vi "Sensor List DAO.vi"(7 "refnum":T1, 8 "error in (no error)":errorcluster, 10 "Sensor List In":refnum<class "Sensor List Class.lvclass">, 11 "Actions":T2) -> (0 "error out":errorcluster, 2 "Sensor List Out":refnum<class "Sensor List Class.lvclass">, 4 "refnum out":T1)   [LabVIEW 2013]
uses:
  Metadata/Persistant DAO Actions.ctl
  Sensor List Class.lvclass
  <vilib>/Utility/config.llb/Config Data RefNum.ctl
  <vilib>/Utility/config.llb/NI_LVConfig.lvlib
panel:
  out "Names":string[](array[string])
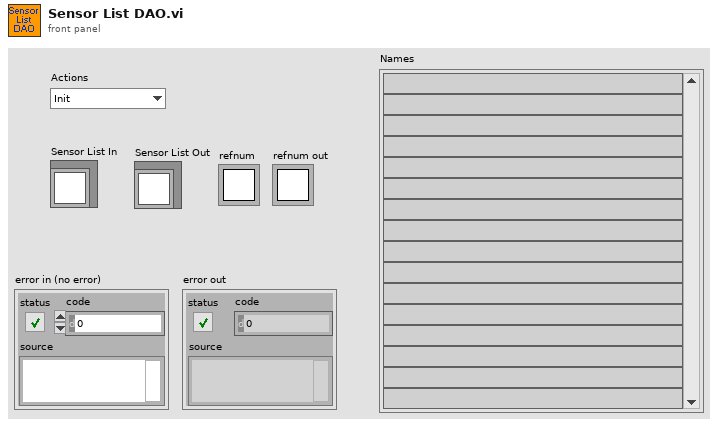
[diagram p1: front panel]
types:
  T1 = typedef "NI_LVConfig.lvlib/Config Data RefNum.ctl" = refnum<k1>
  T2 = typedef "Persistant DAO Actions.ctl" = enum16{"Init", "Get", "Set", "Load", "Save"}
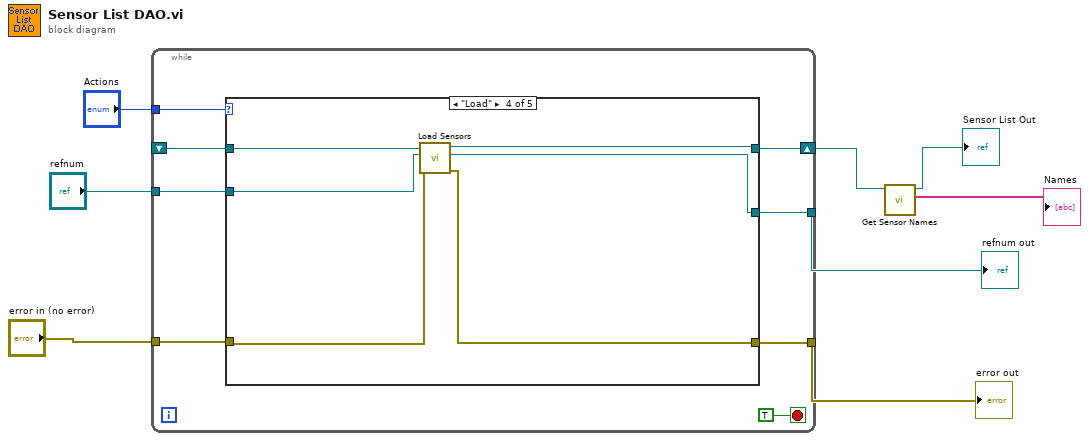
[diagram p0: block diagram]
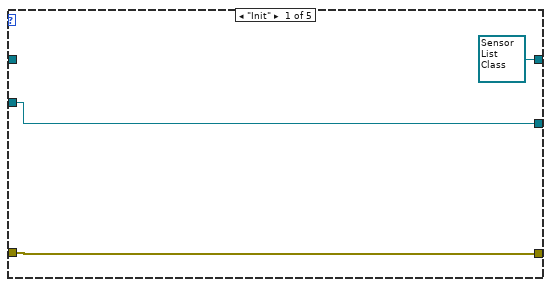
[diagram p2: hidden frame]
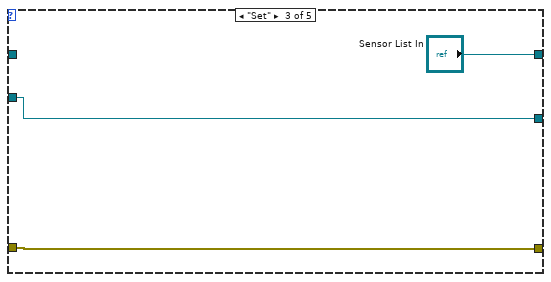
[diagram p4: hidden frame]
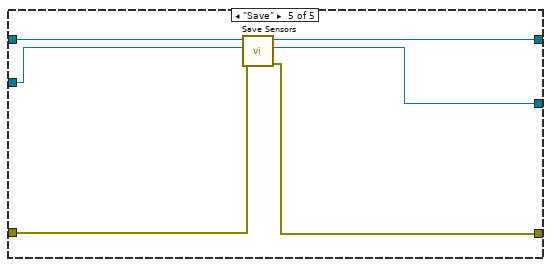
[diagram p5: hidden frame]
diagram:
  n1 = while {
    tunnel: "Actions" -> [w15]
    shift-right: [w14] -> w3
    shift-left: _ -> [w13]
    tunnel: "error in (no error)" -> [w12]
    tunnel: [w11] -> w6
    tunnel: "refnum" -> [w10]
    tunnel: [w9] -> w4
    stop <- TRUE stop-if-true
    n2 = case shown="\"Load\"" w15 {
      tunnel: [refnum<class "Sensor List Class.lvclass"> refnum ("Sensor List In") w22 "Sensor List In" w30 w36] -> w14
      tunnel: w13 -> [_ w22 _ w31 w37]
      tunnel: w12 -> [w18 w21 w24 w29 w35]
      tunnel: [w18 w21 w24 w28 w34] -> w11
      tunnel: w10 -> [w17 w20 w23 w27 w33]
      tunnel: [w17 w20 w23 w26 w32] -> w9
      frame "Init" {
      }
      frame "Get" {
      }
      frame "Set" {
      }
      frame "Load" {
        n3 = call "Load Sensors.vi"("error in (no error)"=w29, "refnum"=w27, "Sensor List Class in"=w31) -> ("error out"=w28:errorcluster, "refnum out"=w26:T1, "Sensor List Class out"=w30:refnum<class "Sensor List Class.lvclass">)  [unwired: 6 in]
      }
      frame "Save" {
        n4 = call "Save Sensors.vi"("error in (no error)"=w35, "refnum"=w33, "Sensor List Class in"=w37) -> ("error out"=w34:errorcluster, "refnum out"=w32:T1, "Sensor List Class out"=w36:refnum<class "Sensor List Class.lvclass">)  [unwired: 6 in]
      }
    }
  }
  "error out" <- w6
  "refnum out" <- w4
  n5 = call "Get Sensor Names.vi"("Sensor List Class in"=w3) -> ("Names"=→"Names":string[], "Sensor List Class out"=→"Sensor List Out":refnum<class "Sensor List Class.lvclass">)  [unwired: 8 in, 1 out]
